vi "WFS Calc Mean Rms Noise.vi"(8 "error in (no error)":errorcluster {"code" format="%.0x"}, 11 "instrument handle":refnum<visa-resource-name>) -> (0 "error out":errorcluster {"code" format="%.0x"}, 1 "Rms":dbl, 2 "Mean":dbl, 3 "instrument handle out":refnum<visa-resource-name>)   [LabVIEW 2020]
doc: "This VI returns the mean average and rms variations of the pixel intensities in ImageBuf.\n\nNote: This VI is not available in Highspeed Mode!"
uses:
  WFS_32.dll
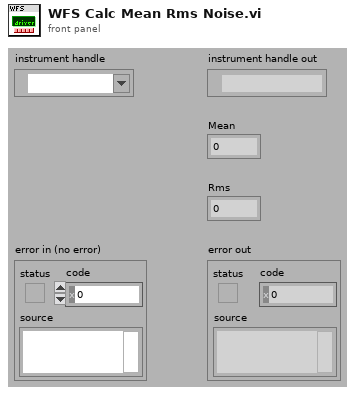
[diagram p1: front panel]
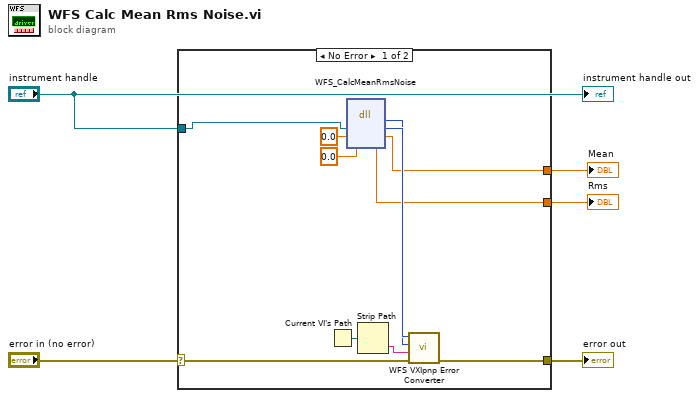
[diagram p0: block diagram]
diagram:
  n1 = case shown="No Error" "error in (no error)" {
    selector: "error in (no error)" -> [w11 w17]
    tunnel: [w10 w17] -> w5
    tunnel: "instrument handle" -> [w15 _]
    tunnel: [w8 _] -> w2
    tunnel: [w6 _] -> w1
    frame No Error {
      n2 = Current VI's Path() -> (path=w16:path)
      n3 = dll-call lib="WFS_*.*" fn="WFS_CalcMeanRmsNoise"("Instrument Handle"=w15, "Mean"=0.0, "Rms"=0.0) -> (w13:i32, "Instrument Handle"=w14:u32, "Mean"=w8:dbl, "Rms"=w6:dbl)  [unwired: 3 in, 2 out]
      n4 = Strip Path(path=w16) -> (name=w12:string)  [unwired: 1 out]
      n5 = call "WFS VXIpnp Error Converter.vi"("error in (no error)"=w11, "Name Of VI (\"\")"=w12, "CVI Error Code (0)"=w13, "instrument handle"=w14) -> ("error out"=w10:errorcluster)  [unwired: 6 in, 1 out]
    }
    frame Error {
    }
  }
  "error out" <- w5
  "Mean" <- w2
  "Rms" <- w1
  "instrument handle out" <- "instrument handle"
